vi "Lab_Temp_PID.vi"(1 "Present Value":dbl=15.0 format="%.2f", 2 "Previous Control Sum":dbl format="%.2f", 3 "Setpoint":dbl=15.0 format="%.2f") -> (0 "Dem Output":dbl format="%.2f")   [LabVIEW 2010]
uses:
  <vilib>/Analysis/NI_AALPro.lvlib
panel:
  in  "O/P deadband":dbl=0.5 format="%.2f"
  in  "Kp Deadband":dbl format="%.2f"
  in  "Derivative History":i32=20
  out "deadbanded error":dbl format="%.2f"
  in  "P":bool=TRUE
  in  "D":bool=TRUE
  in  "I":bool=TRUE
  out "Waveform Chart":T1(graph)
  in  "Manual Demand":dbl min=0.0 max=100.0 format="%.2f"
  in  "Manual Override":bool
  out "Control Sum":dbl format="%.2f"
  out "Derivative Term":dbl format="%.2f"
  out "Integral Term":dbl format="%.2f"
  out "error differential":dbl format="%.5f"
  out "error integral":dbl format="%.2f"
  out "Proportional Term":dbl format="%.2f"
  in  "Kd":dbl=50.0 format="%.2f"
  in  "Ki":dbl=40.0 format="%.2f"
  in  "Kp":dbl=30.0 format="%.2f"
  out "error":dbl format="%.2f"
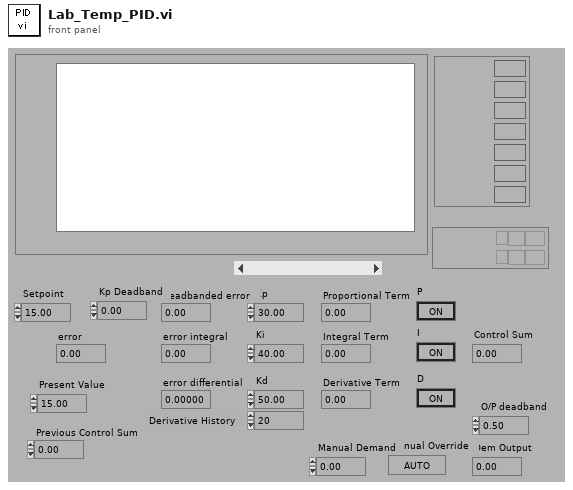
[diagram p1: front panel]
types:
  T1 = cluster{"Setpoint":dbl, "Present Value":dbl, "Proportional Term":dbl, "Integral Term":dbl, "Derivative Term":dbl, "Control Sum":dbl, "Dem Output":dbl}
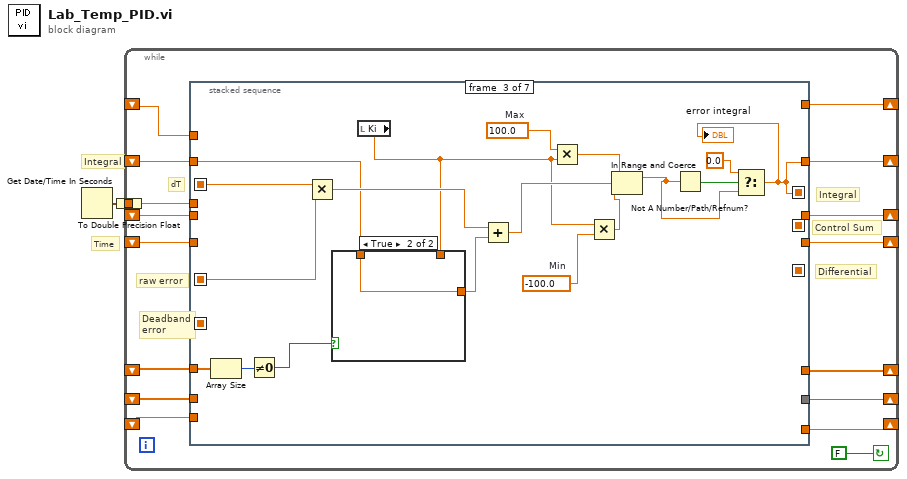
[diagram p0: block diagram]
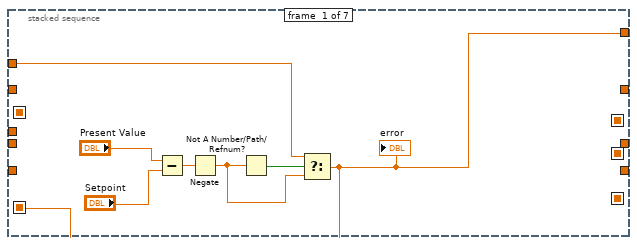
[diagram p2: hidden frame]
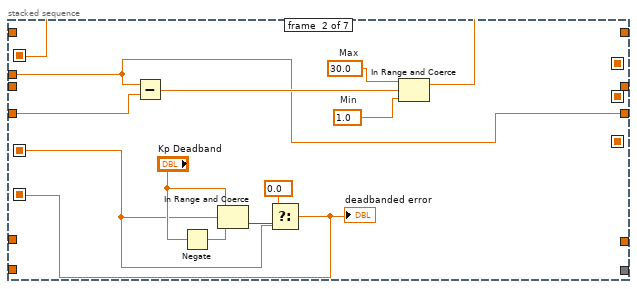
[diagram p3: hidden frame]
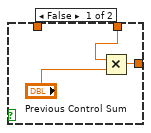
[diagram p4: hidden frame]
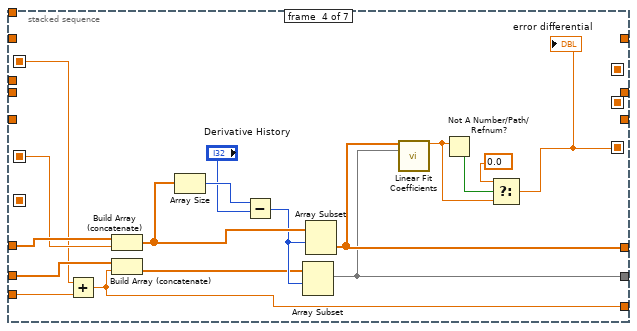
[diagram p5: hidden frame]
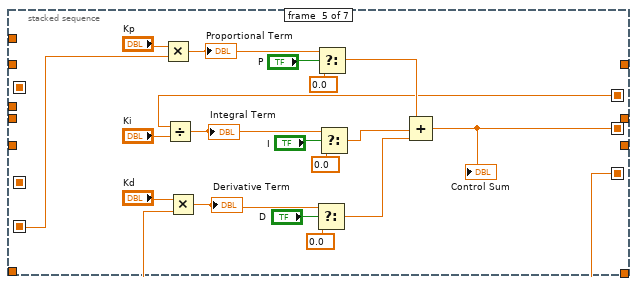
[diagram p6: hidden frame]
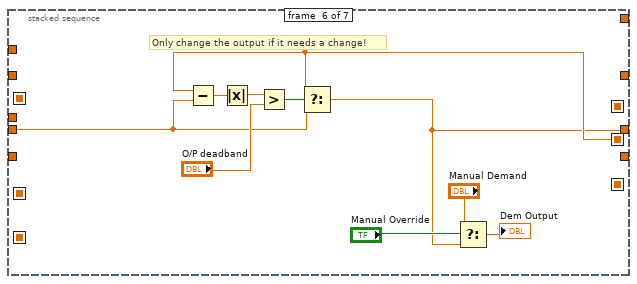
[diagram p7: hidden frame]
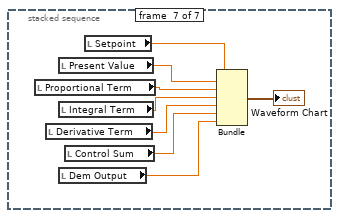
[diagram p8: hidden frame]
diagram:
  # "Integral"
  # "Time"
  n1 = Get Date/Time In Seconds() -> (seconds since 1Jan1904=w1:timestamp)
  n2 = To Double Precision Float(number=w1) -> (double precision float=w2:dbl)
  n3 = while {
    shift-left: _ -> [w5]
    shift-right: [w4] -> _
    shift-left: _ -> [w7]
    shift-right: [w6] -> _
    shift-left: _ -> [w9]
    shift-right: [w8] -> _
    tunnel: w2 -> [w14]
    shift-left: _ -> [w11]
    shift-right: [w10] -> _
    shift-left: _ -> [w13]
    shift-right: [w12] -> _
    shift-left: _ -> [w15]
    shift-right: [w16] -> _
    shift-left: _ -> [w18]
    shift-right: [w17] -> _
    stop <- FALSE continue-if-true
    # "Control Sum"
    # "raw error"
    # "Differential"
    # "Integral"
    # "Deadband\nerror"
    # "dT"
    n4 = stacked-sequence {
      seq-local: [_ w26 _ _ _ _ _] -> [_ _ w55 w62 _ _ _]
      seq-local: [_ w35 _ _ _ _ _] -> [_ _ _ _ w80 _ _]
      seq-local: [_ _ _ w67 _ _ _] -> [_ _ _ _ w79 _ _]
      seq-local: [_ _ w41 _ _ _ _] -> [_ _ _ _ w78 _ _]
      seq-local: [w20 _ _ _ _ _ _] -> [_ w27 w51 w68 _ _ _]
      seq-local: [_ _ _ _ w83 _ _] -> [_ _ _ _ _ w99 _]
      tunnel: w18 -> [_ w32 _ _ _ _ _]
      tunnel: [_ w30 _ _ _ _ _] -> w17
      tunnel: [_ _ w41 _ _ _ _] -> w16
      tunnel: w15 -> [_ _ w45 _ _ _ _]
      tunnel: w14 -> [_ w30 _ _ _ _ _]
      tunnel: w13 -> [_ _ w50 w76 _ _ _]
      tunnel: [_ _ _ w69 _ _ _] -> w12
      tunnel: w11 -> [_ _ _ w75 _ _ _]
      tunnel: [_ _ _ w66 _ _ _] -> w10
      tunnel: w9 -> [_ _ _ _ _ w97 _]
      tunnel: [_ _ _ _ _ w96 _] -> w8
      tunnel: w7 -> [_ _ _ w61 _ _ _]
      tunnel: [_ _ _ w60 _ _ _] -> w6
      tunnel: w5 -> [w22 _ _ _ _ _ _]
      tunnel: [w20 _ _ _ _ _ _] -> w4
      frame #0 {
        n5 = Subtract(x="Present Value", y="Setpoint") -> (x-y=w21:dbl)
        n6 = Negate(x=w21) -> (-x=w19:dbl)
        n7 = Not A Number/Path/Refnum?(number/path/refnum=w19) -> (NaN/Path/Refnum?=w23:bool)
        n8 = Select(t=w22, s=w23, f=w19) -> (s? t:f=w20:dbl)
        "error" <- w20
      }
      frame #1 {
        w33 = 1.0  # Min
        w34 = 30.0  # Max
        n9 = Subtract(x=w30, y=w32) -> (x-y=w31:dbl)
        n10 = Negate(x="Kp Deadband") -> (-x=w29:dbl)
        n11 = In Range and Coerce(upper limit="Kp Deadband", x=w27, lower limit=w29) -> (In Range?=w36:bool)  [unwired: 1 out]
        n12 = Select(t=0.0, s=w36, f=w27) -> (s? t:f=w35:dbl)
        "deadbanded error" <- w35
        n13 = In Range and Coerce(upper limit=w34, x=w31, lower limit=w33) -> (coerced(x)=w26:dbl)  [unwired: 1 out]
      }
      frame #2 {
        w40 = -100.0  # Min
        w54 = 100.0  # Max
        n14 = Array Size(array=w50) -> (size(s)=w49:i32)
        n15 = Not Equal To 0?(x=w49) -> (x != 0?=w47:bool)
        n16 = Multiply(x=w55, y=w51) -> (x*y=w48:dbl)
        n17 = local read "Ki"() -> (w38:dbl)
        n18 = case shown="True" w47 {
          tunnel: [w56 w59] -> w46
          tunnel: w45 -> [_ w59]
          tunnel: w38 -> [w58 _]
          frame False {
            n19 = Multiply(x=w58, y="Previous Control Sum") -> (x*y=w56:dbl)
          }
          frame True {
          }
        }
        n20 = Add(x=w48, y=w46) -> (x+y=w52:dbl)
        n21 = Multiply(x=w54, y=w38) -> (x*y=w53:dbl)
        n22 = Multiply(x=w38, y=w40) -> (x*y=w39:dbl)
        n23 = In Range and Coerce(upper limit=w53, x=w52, lower limit=w39) -> (coerced(x)=w43:dbl)  [unwired: 1 out]
        n24 = Not A Number/Path/Refnum?(number/path/refnum=w43) -> (NaN/Path/Refnum?=w44:bool)
        n25 = Select(t=0.0, s=w44, f=w43) -> (s? t:f=w41:dbl)
        "error integral" <- w41
      }
      frame #3 {
        n26 = Add(x=w62, y=w61) -> (x+y=w60:dbl)
        n27 = Build Array (concatenate)(w76, w68) -> (w72:dbl[])
        n28 = Build Array (concatenate)(w75, w60) -> (w70:dbl[])
        n29 = Array Size(array=w72) -> (size(s)=w74:i32)
        n30 = Subtract(x=w74, y="Derivative History") -> (x-y=w71:i32)
        n31 = Array Subset(array=w70, index=w71) -> (w66:dbl[])  [unwired: 1 in]
        n32 = Array Subset(array=w72, index=w71) -> (w69:dbl[])  [unwired: 1 in]
        n33 = call <vilib>:"Linear Fit Coefficients.vi"("Y"=w69, "X"=w66) -> ("slope"=w63:dbl)  [unwired: 3 in, 10 out]
        n34 = Not A Number/Path/Refnum?(number/path/refnum=w63) -> (NaN/Path/Refnum?=w65:bool)
        n35 = Select(t=0.0 ("f"), s=w65, f=w63) -> (s? t:f=w67:dbl)
        "error differential" <- w67
      }
      frame #4 {
        n36 = Multiply(x="Kp", y=w80) -> (x*y=w93:dbl)
        "Proportional Term" <- w93
        n37 = Divide(x=w78, y="Ki") -> (x/y=w84:dbl)
        "Integral Term" <- w84
        n38 = Multiply(x="Kd", y=w79) -> (x*y=w85:dbl)
        "Derivative Term" <- w85
        n39 = Select(t=w85, s="D", f=0.0) -> (s? t:f=w87:dbl)
        n40 = Select(t=w93, s="P", f=0.0) -> (s? t:f=w94:dbl)
        n41 = Select(t=w84, s="I", f=0.0) -> (s? t:f=w86:dbl)
        n42 = Compound Arithmetic op=ADD(w94, w86, w87) -> (w83:dbl)
        "Control Sum" <- w83
      }
      frame #5 {
        # "Only change the output if it needs a change!"
        n43 = Subtract(x=w99, y=w97) -> (x-y=w102:dbl)
        n44 = Absolute Value(x=w102) -> (abs(x)=w101:dbl)
        n45 = Greater?(x=w101, y="O/P deadband") -> (0:w100:bool)
        n46 = Select(t=w99, s=w100, f=w97) -> (s? t:f=w96:dbl)
        n47 = Select(t="Manual Demand", s="Manual Override", f=w96) -> (s? t:f=→"Dem Output":dbl)
      }
      frame #6 {
        n48 = local read "Proportional Term"() -> (w109:dbl)
        n49 = local read "Derivative Term"() -> (w111:dbl)
        n50 = local read "Present Value"() -> (w108:dbl)
        n51 = local read "Integral Term"() -> (w110:dbl)
        n52 = local read "Dem Output"() -> (w113:dbl)
        n53 = local read "Control Sum"() -> (w112:dbl)
        n54 = local read "Setpoint"() -> (w107:dbl)
        n55 = Bundle("Setpoint"=w107, "Present Value"=w108, "Proportional Term"=w109, "Integral Term"=w110, "Derivative Term"=w111, "Control Sum"=w112, "Dem Output"=w113) -> (→"Waveform Chart":T1)  [unwired: 1 out]
      }
    }
  }
